vi "Build notes string.vi"(10 "Weekday filter":T2, 11 "Quarter Filter":T1 {"month ring" items=["Jan", "Feb", "Mar", "Apr", "May", "Jun", "Jul", "Ago", "Set", "Oct", "Nov", "Dec"]}) -> (3 "spreadsheet string 2":string)   [LabVIEW 2018]
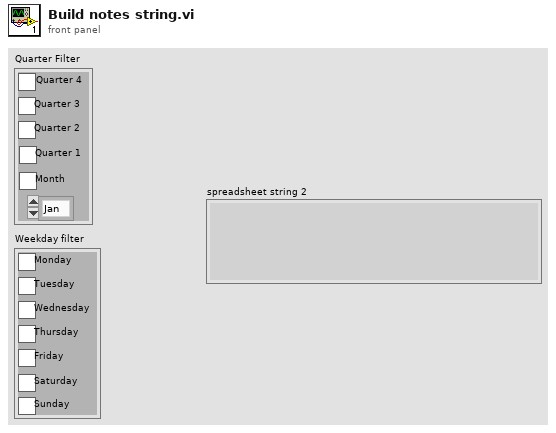
[diagram p1: front panel]
types:
  T1 = cluster{"Q1 3":bool, "Q2 2":bool, "Q3 2":bool, "Q4 2":bool, "Q1 4":bool, "month ring":u16}
  T2 = cluster{"Monday":bool, "Tuesday":bool, "Wednesday":bool, "Thursday":bool, "Friday":bool, "Saturday":bool, "Sunday":bool}
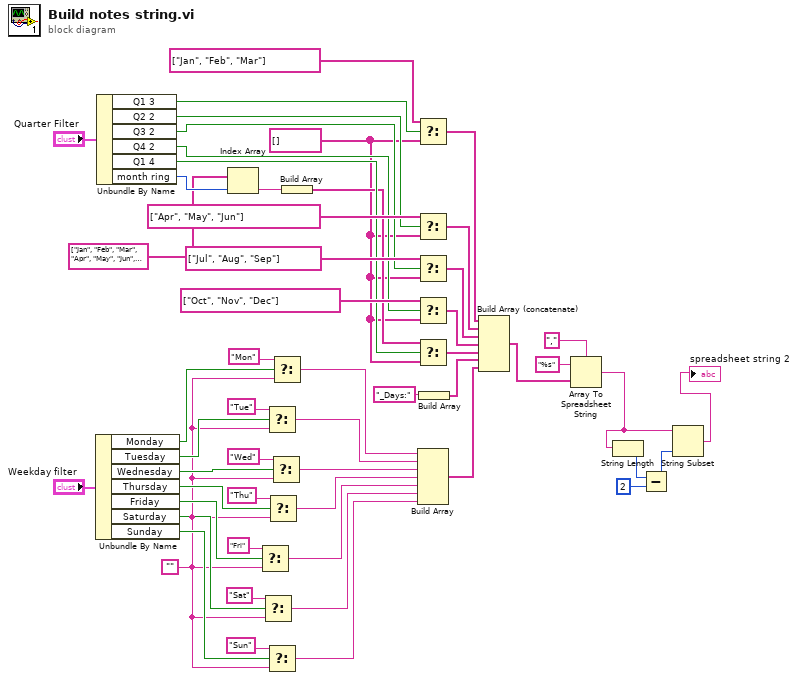
[diagram p0: block diagram]
diagram:
  w13 = ""
  w36 = string[] []
  n1 = Unbundle By Name("Weekday filter") -> ("Monday"=w34:bool, "Tuesday"=w26:bool, "Wednesday"=w25:bool, "Thursday"=w24:bool, "Friday"=w23:bool, "Saturday"=w22:bool, "Sunday"=w21:bool)
  n2 = Unbundle By Name("Quarter Filter") -> ("Q1 3"=w42:bool, "Q2 2"=w44:bool, "Q3 2"=w45:bool, "Q4 2"=w46:bool, "Q1 4"=w40:bool, "month ring"=w39:u16)
  n3 = Index Array(array=string[] ["Jan", "Feb", "Mar", "Apr", "May", "Jun", "Jul", "Aug", "Sep", "Oct", "Nov", "Dec"] ("appended array"), index=w39) -> (element=w38:string)
  n4 = Select(t="Fri" ("String"), s=w23, f=w13) -> (s? t:f=w16:string)
  n5 = Select(t="Sat" ("String"), s=w22, f=w13) -> (s? t:f=w15:string)
  n6 = Select(t="Tue" ("String"), s=w26, f=w13) -> (s? t:f=w19:string)
  n7 = Select(t="Sun" ("String"), s=w21, f=w13) -> (s? t:f=w14:string)
  n8 = Select(t="Thu" ("String"), s=w24, f=w13) -> (s? t:f=w17:string)
  n9 = Select(t="Wed" ("String"), s=w25, f=w13) -> (s? t:f=w18:string)
  n10 = Select(t="Mon" ("String"), s=w34, f=w13) -> (s? t:f=w20:string)
  n11 = Build Array(w38) -> (w37:string[])
  n12 = Select(t=string[] ["Jan", "Feb", "Mar"], s=w42, f=w36) -> (s? t:f=w50:string[])
  n13 = Select(t=string[] ["Apr", "May", "Jun"], s=w44, f=w36) -> (s? t:f=w51:string[])
  n14 = Select(t=string[] ["Jul", "Aug", "Sep"], s=w45, f=w36) -> (s? t:f=w52:string[])
  n15 = Select(t=string[] ["Oct", "Nov", "Dec"], s=w46, f=w36) -> (s? t:f=w41:string[])
  n16 = Select(t=w37, s=w40, f=w36) -> (s? t:f=w35:string[])
  n17 = Build Array(w20, w19, w18, w17, w16, w15, w14) -> (w8:string[])
  n18 = Build Array("_Days:" ("String")) -> (w6:string[])
  n19 = Build Array (concatenate)(w50, w51, w52, w41, w35, w6, w8) -> (w9:string[])
  n20 = Array To Spreadsheet String(delimiter (Tab)=",", array=w9, 3:"%s" ("format string")) -> (spreadsheet string=w2:string)
  n21 = String Length(string=w2) -> (length=w5:i32)
  n22 = Subtract(x=w5, y=2) -> (x-y=w3:i32)
  n23 = String Subset(string=w2, length (rest)=w3) -> (substring=→"spreadsheet string 2":string)  [unwired: 1 in]
